vi "Calling-Python-Script.vi"() -> ()   [LabVIEW 2012]
panel:
  in  "Path to Python.exe":path=path "C:/Python26/python.exe"
  out "Raw Python String Output":string
  out "error out":errorcluster
  out "Standard Error":string
  out "Return Code":i32
  # "1. Inputs - Set before running VI"
  # "2. Outputs"
  # "3. Errors - Both Standard and LabVIEW"
  # "A + B ="
  # "This VI sends inputs to a simple Python script, and returns its output.\n\nSee block diagram for code and comments"
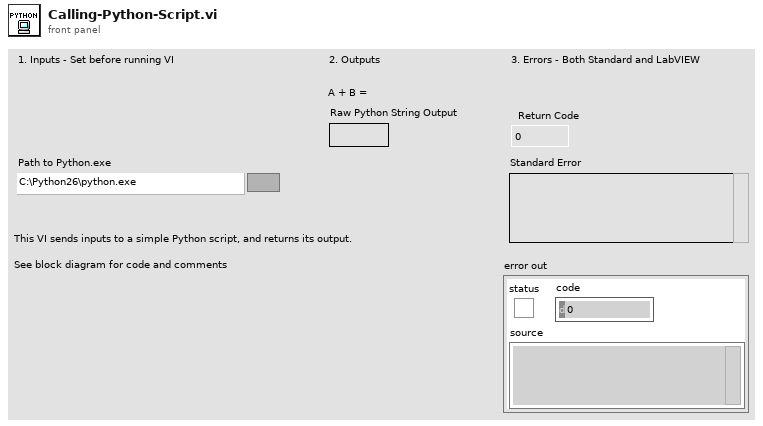
[diagram p1: front panel]
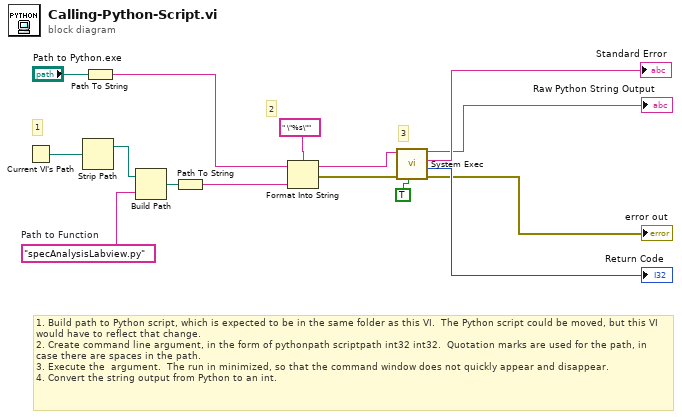
[diagram p0: block diagram]
diagram:
  w12 = "specAnalysisLabview.py"  # Path to Function
  # "1. Build path to Python script, which is expected to be in the same folder as this VI.  The Python script could be moved, but this VI would have to reflect that change.\n2. Create command line argument, in the form of pythonpath scriptpath int32 int32.  Quotation marks are used for the path, in case there are spaces in the path.\n3. Execute the  argument.  The run in minimized, so that the command window does not quickly appear and disappear.\n4. Convert the string output from Python to an int."
  # "3"
  # "2"
  # "1"
  n1 = Current VI's Path() -> (path=w6:path)
  n2 = Strip Path(path=w6) -> (stripped path=w3:path)  [unwired: 1 out]
  n3 = Path To String(path="Path to Python.exe") -> (string=w5:string)
  n4 = Build Path(base path=w3, name or relative path=w12) -> (appended path=w10:path)
  n5 = Path To String(path=w10) -> (string=w11:string)
  n6 = Format Into String "Format Into String"(format string=" \"%s\"", initial string=w5, w11) -> (resulting string=w9:string, error out=w7:errorcluster)  [unwired: 1 in]
  n7 = call <vilib>:"System Exec.vi"("run minimized? (F)"=TRUE, "error in (no error)"=w7, "command line"=w9) -> ("error out"=→"error out":errorcluster, "return code"=→"Return Code":i32, "standard error"=→"Standard Error":string, "standard output"=→"Raw Python String Output":string)  [unwired: 5 in]
